vi "GVSGet Numeric Reference.vi"(10 "Label Name":string, 11 "VI Refnum":refnum<vi>) -> (1 "Boolean":bool, 2 "Numeric Ref Out":refnum<vi>, 3 "VI Refnum Out":refnum<vi>)   [LabVIEW 2013]
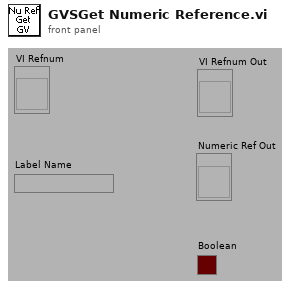
[diagram p1: front panel]
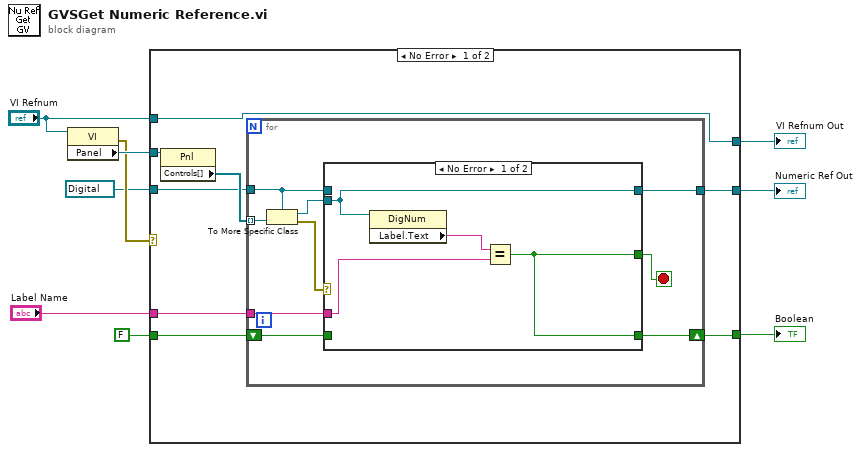
[diagram p0: block diagram]
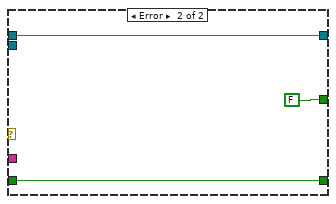
[diagram p2: hidden frame]
diagram:
  n1 = property class="VI"(reference="VI Refnum") -> (error out=w6:errorcluster, "Panel"=w8:refnum<vi>)  [unwired: 1 in, 1 out]
  n2 = case shown="No Error" w6 {
    tunnel: "Label Name" -> [w17 _]
    tunnel: w8 -> [w16 _]
    tunnel: "VI Refnum" -> [w12 w35]
    tunnel: refnum<vi> refnum ("Numeric") -> [w14 w34]
    tunnel: [w13 w34] -> w4
    tunnel: [w12 w35] -> w3
    tunnel: FALSE ("Boolean") -> [w11 w36]
    tunnel: [w10 w36] -> w1
    frame No Error {
      n3 = property class="Pnl"(reference=w16) -> ("Controls[]"=w15:refnum<vi>[])  [unwired: 1 in, 2 out]
      n4 = for {
        tunnel: w15 -> [w26] mode=indexing
        tunnel: [w22] -> w13
        tunnel: w17 -> [w21]
        tunnel: w14 -> [w20]
        shift-right: [w18] -> w10
        shift-left: w11 -> [w19]
        stop <- w23 stop-if-true
        n5 = To More Specific Class(target class=w20, reference=w26) -> (specific class reference=w24:refnum<vi>, error out=w25:errorcluster)  [unwired: 1 in]
        n6 = case shown="No Error" w25 {
          tunnel: w24 -> [w28 _]
          tunnel: [w27 FALSE] -> w23
          tunnel: [w28 w32] -> w22
          tunnel: w21 -> [w29 _]
          tunnel: w20 -> [_ w32]
          tunnel: w19 -> [_ w31]
          tunnel: [w27 w31] -> w18
          frame No Error {
            n7 = property class="DigNum"(reference=w28) -> ("Label.Text"=w30:string)  [unwired: 1 in, 2 out]
            n8 = Equal?(x=w30, y=w29) -> (x = y?=w27:bool)
          }
          frame Error {
          }
        }
      }
    }
    frame Error {
    }
  }
  "Boolean" <- w1
  "VI Refnum Out" <- w3
  "Numeric Ref Out" <- w4
